vi "Fusion Wavelets (Basic).vi"() -> (6 "Fusion Method":cluster{"approximation":u16, "detail":u16}={"approximation"=2, "detail"=2} {"detail" items=["Max", "Min", "Mean", "Image 1", "Image 2"]; "approximation" items=["Max", "Min", "Mean", "Image 1", "Image 2"]})   [LabVIEW 2023]
doc: "Computes the detail and approximation coefficients of two images using the WA Discrete Wavelet Transform VI, merges the resulting coefficients, and computes the fusion image using the WA Inverse Discrete Wavelet Transform VI."
uses:
  <vilib>/addons/Wavelet Analysis/discrete wavelet transform.llb/WA 2D Discrete Wavelet Transform.vi
  <vilib>/addons/Wavelet Analysis/discrete wavelet transform.llb/WA Inverse 2D Discrete Wavelet Transform.vi
  <vilib>/addons/_Advanced Signal Processing/NI_AdvSigProcWA.lvlib
panel:
  in  "Image":bool
  out "Image 2 (High Energy)":T1(plugin-control)
  out "Image 1 (Low energy)":T1(plugin-control)
  in  "Wavelet":u16(ring) items=["db02"=0, "db03"=1, "db04"=2, "db05"=3, "db06"=4, "db07"=5, "db08"=6, "db09"=7, "db10"=8, "db11"=9, "db12"=10, "db13"=11, "db14"=12, "Haar"=13, "bior1_3"=14, "bior1_5"=15, "bior2_2"=16, "bior2_4"=17, "bior2_6"=18, "bior2_8"=19, "bior3_1"=20, "bior3_3"=21, "bior3_5"=22, "bior3_7"=23, "bior3_9"=24, "bior4_4 (FBI)"=25, "bior5_5"=38, "bior6_8"=39, "coif1"=26, "coif2"=27, "coif3"=28, "coif4"=29, "coif5"=30, "sym2"=31, "sym3"=32, "sym4"=33, "sym5"=34, "sym6"=35, "sym7"=36, "sym8"=37]
  out "Fusion":T1(plugin-control)
  # "Images Fusion using Wavelets"
  # "This is an attempt to combine two shots taken at different energies, where one is \"underexposured\" and the other one \"overexposured\"\nto get overall better CNR for thin and thick areas in single image."
  # "1"
  # "2"
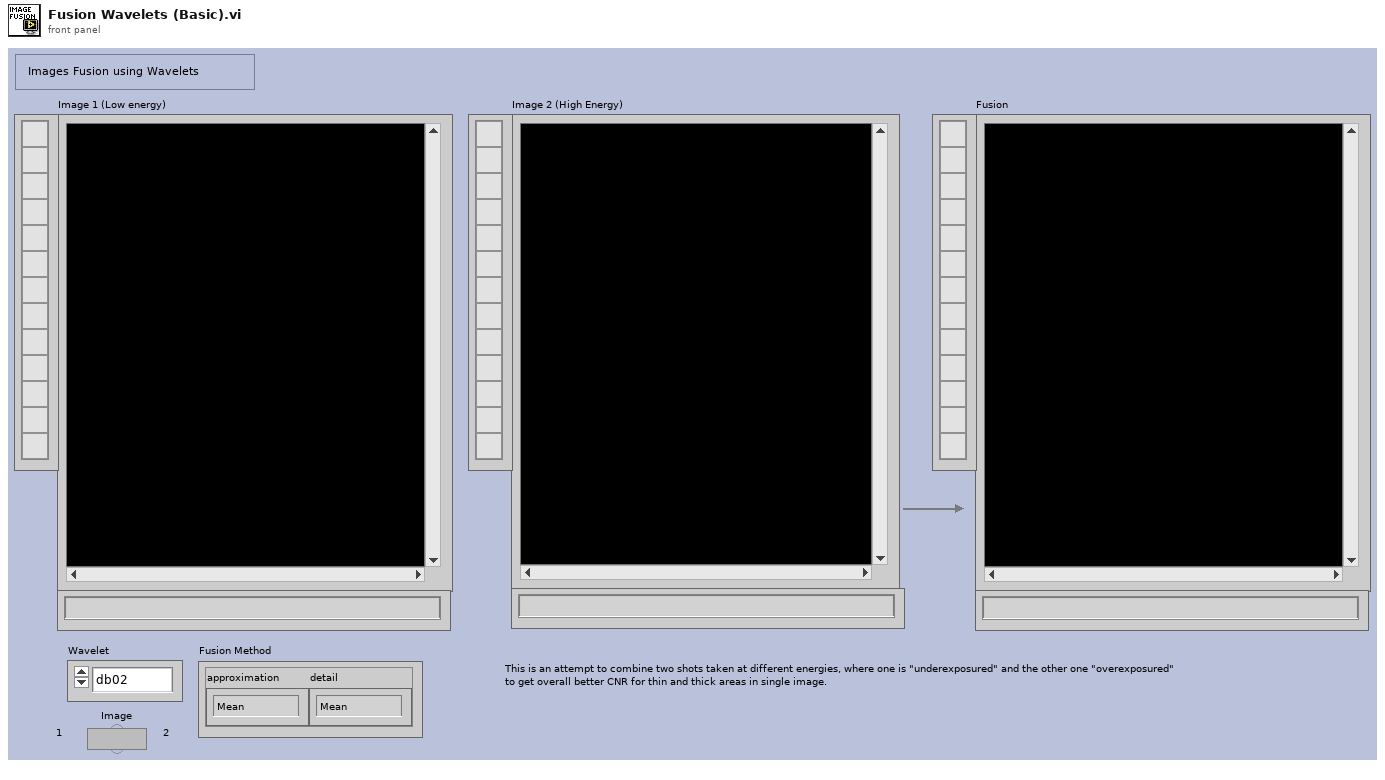
[diagram p1: front panel]
types:
  T1 = typedef "IMAQ Image.ctl" = refnum<image>
  T2 = typedef "Image Type" = u32
  T3 = cluster{"low_low":dbl[][], "low_high":dbl[][], "high_low":dbl[][], "high_high":dbl[][]}[]
  T4 = cluster{"low_low":dbl[][], "low_high":dbl[][], "high_low":dbl[][], "high_high":dbl[][]}
  T5 = cluster{"low_low":dbl[][], "Fusion Coef":dbl[][], "Fusion Coef":dbl[][], "Fusion Coef":dbl[][]}
  T6 = cluster{"low_low":dbl[][], "Fusion Coef":dbl[][], "Fusion Coef":dbl[][], "Fusion Coef":dbl[][]}[]
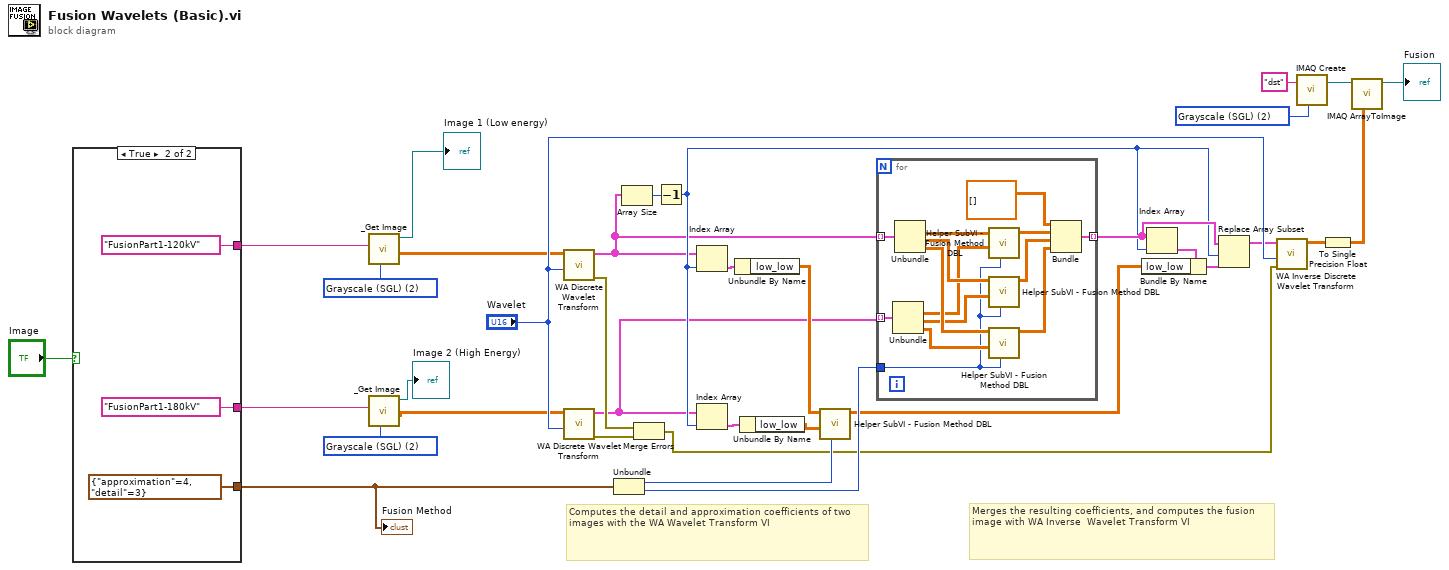
[diagram p0: block diagram]
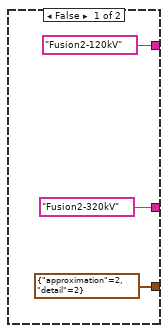
[diagram p2: hidden frame]
diagram:
  w30 = T2 2 items=["Grayscale (U8)", "Grayscale (I16)", "Grayscale (SGL)", "Complex (CSG)", "RGB (U32)", "HSL (U32)", "RGB (U64)", "Grayscale (U16)"] ("Image Type (U16)")
  w32 = T2 2 items=["Grayscale (U8)", "Grayscale (I16)", "Grayscale (SGL)", "Complex (CSG)", "RGB (U32)", "HSL (U32)", "RGB (U64)", "Grayscale (U16)"] ("Image Type")
  w35 = T2 2 items=["Grayscale (U8)", "Grayscale (I16)", "Grayscale (SGL)", "Complex (CSG)", "RGB (U32)", "HSL (U32)", "RGB (U64)", "Grayscale (U16)"] ("Image Type (U16)")
  # "Merges the resulting coefficients, and computes the fusion image with WA Inverse  Wavelet Transform VI"
  # "Computes the detail and approximation coefficients of two images with the WA Wavelet Transform VI"
  n1 = case shown="True" "Image" {
    tunnel: ["Fusion2-120kV" ("Image Name") "FusionPart1-120kV" ("Image Name")] -> w4
    tunnel: ["Fusion2-320kV" ("Image Name") "FusionPart1-180kV" ("Image Name")] -> w3
    tunnel: [cluster{"approximation":u16, "detail":u16} {"approximation"=2, "detail"=2} ("Fusion Method") cluster{"approximation":u16, "detail":u16} {"approximation"=4, "detail"=3} ("Fusion Method")] -> w2
    frame False {
    }
    frame True {
    }
  }
  "Fusion Method" <- w2
  n2 = call "_Get Image.vi"("Image Type (U16)"=w35, "Image Name"=w4) -> ("Image Pixels (Float)"=w6:dbl[][], "Image Out"=→"Image 1 (Low energy)":T1)  [unwired: 6 in, 2 out]
  n3 = call "_Get Image.vi"("Image Type (U16)"=w30, "Image Name"=w3) -> ("Image Pixels (Float)"=w5:dbl[][], "Image Out"=→"Image 2 (High Energy)":T1)  [unwired: 6 in, 2 out]
  n4 = call-poly <vilib>:"WA Discrete Wavelet Transform.vi"("wavelet"="Wavelet", "signal"=w6) -> ("error out"=w16:errorcluster, "DWT coef"=w13:T3)  [unwired: 8 in]
  n5 = call-poly <vilib>:"WA Discrete Wavelet Transform.vi"("wavelet"="Wavelet", "signal"=w5) -> ("error out"=w15:errorcluster, "DWT coef"=w12:T3)  [unwired: 8 in]
  n6 = Unbundle(w2) -> ("approximation"=w23:u16, "detail"=w22:u16)
  n7 = Array Size(array=w13) -> (size(s)=w28:i32)
  n8 = Merge Errors(w16, w15) -> (w14:errorcluster)
  n9 = Decrement(x=w28) -> (x-1=w17:i32)
  n10 = Index Array(array=w13, index=w17) -> (element=w27:T4)
  n11 = Index Array(array=w12, index=w17) -> (element=w26:T4)
  n12 = Unbundle By Name(w27) -> ("low_low"=w25:dbl[][])
  n13 = Unbundle By Name(w26) -> ("low_low"=w24:dbl[][])
  n14 = call "Helper SubVI - Fusion Method DBL.vi"("method"=w23, "Coef 2"=w24, "Coef 1"=w25) -> ("Fusion Coef"=w20:dbl[][])  [unwired: 8 in]
  n15 = for {
    tunnel: w13 -> [w55] mode=indexing
    tunnel: w12 -> [w54] mode=indexing
    tunnel: w22 -> [w47]
    tunnel: [w43] -> w19 mode=indexing
    n16 = Unbundle(w54) -> ("low_high"=w50:dbl[][], "high_low"=w49:dbl[][], "high_high"=w48:dbl[][])  [unwired: 1 out]
    n17 = Unbundle(w55) -> ("low_high"=w53:dbl[][], "high_low"=w52:dbl[][], "high_high"=w51:dbl[][])  [unwired: 1 out]
    n18 = call "Helper SubVI - Fusion Method DBL.vi"("method"=w47, "Coef 2"=w50, "Coef 1"=w53) -> ("Fusion Coef"=w46:dbl[][])  [unwired: 8 in]
    n19 = call "Helper SubVI - Fusion Method DBL.vi"("method"=w47, "Coef 2"=w49, "Coef 1"=w52) -> ("Fusion Coef"=w45:dbl[][])  [unwired: 8 in]
    n20 = call "Helper SubVI - Fusion Method DBL.vi"("method"=w47, "Coef 2"=w48, "Coef 1"=w51) -> ("Fusion Coef"=w44:dbl[][])  [unwired: 8 in]
    n21 = Bundle("low_low"=dbl[][] [], "Fusion Coef"=w46, "Fusion Coef"=w45, "Fusion Coef"=w44) -> (w43:T5)  [unwired: 1 out]
  }
  n22 = Index Array(array=w19, index=w17) -> (element=w21:T5)
  n23 = Bundle By Name(cluster=w21, "low_low"=w20) -> (w18:T5)
  n24 = Replace Array Subset(array=w19, new element=w18, index=w17) -> (w11:T6)
  n25 = call-poly <vilib>:"WA Inverse Discrete Wavelet Transform.vi"("error in (no error)"=w14, "wavelet"="Wavelet", "DWT coef"=w11) -> ("signal"=w34:dbl[][])  [unwired: 7 in, 1 out]
  n26 = call "IMAQ Create"("Image Name"="dst", "Image Type"=w32) -> ("New Image"=w31:T1)  [unwired: 3 in, 1 out]
  n27 = To Single Precision Float(number=w34) -> (single precision float=w10:sgl[][])
  n28 = call "IMAQ ArrayToImage"("Image Pixels (Float)"=w10, "Image"=w31) -> ("Image Out"=→"Fusion":T1)  [unwired: 8 in, 1 out]
